vi "未命名 1.vi"() -> ()   [LabVIEW 2013]
panel:
  out "PF(2)":i32 format="%x"
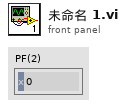
[diagram p1: front panel]
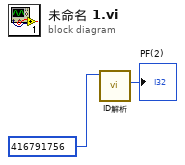
[diagram p0: block diagram]
diagram:
  n1 = call "ID解析.vi"("ID"=u32 416791756) -> ("PF(2)"=→"PF(2)":i32)  [unwired: 10 out]
